vi "OptimizedFPGA_SPI_ReadAuto.vi"(8 "error in (no error)":errorcluster, 9 "Bytes per Sample":u32, 10 "Samples to Read":u32) -> (0 "error out":errorcluster, 2 "Data":u8[][](array[numeric]))   [LabVIEW 2017]
uses:
  <vilib>/Utility/error.llb/Error Cluster From Error Code.vi
  <vilib>/rvi/errors/niLvFpgaAdjustHostInterfaceError.vi
  <vilib>/rvi/interface/nirviMethod/nirviMethod.xnode
  <vilib>/Rock Robotics/SystemInterfaces/System/FPGA_SystemFRC FPGA Ref.ctl
  <vilib>/FPGAPlugInAG/Dynamic/niLvFpga_ReadFifo_Dynamic.vi
  <vilib>/rvi/errors/niLvFpgaMergeErrorWithErrorCode.vi
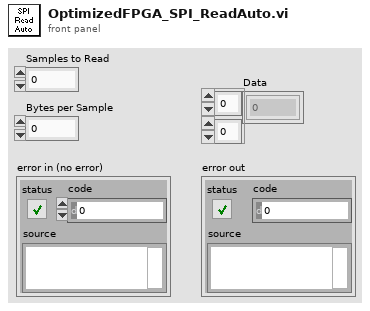
[diagram p1: front panel]
types:
  T1 = typedef "FPGA_SystemFRC FPGA Ref.ctl" = refnum<k20>
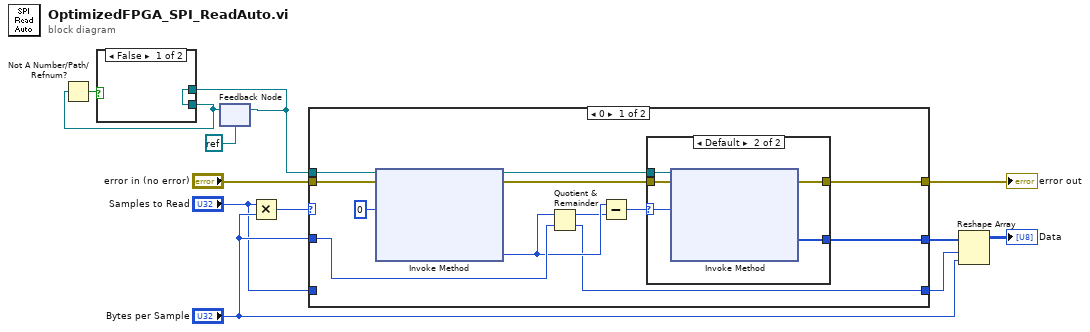
[diagram p0: block diagram]
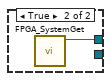
[diagram p2: hidden frame]
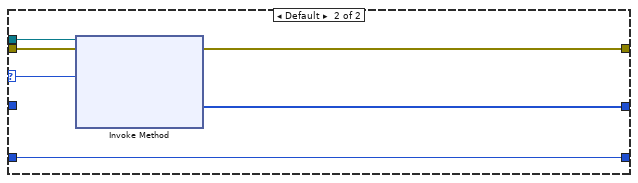
[diagram p4: hidden frame]
diagram:
  n1 = feedback #1(refnum<k0> refnum) -> (w2:T1)
  n2 = Not A Number/Path/Refnum?(number/path/refnum=w2) -> (NaN/Path/Refnum?=w3:bool)
  n3 = case shown="False" w3 {
    tunnel: [w13 w14] -> w4
    tunnel: w2 -> [w13 _]
    frame False {
    }
    frame True {
      n4 = call <vilib>:"FPGA_SystemGet.vi"() -> ("FRC FPGA Ref"=w14:T1)  [unwired: 11 in]
    }
  }
  n5 = feedback-in #1(w4) -> ()
  n6 = Multiply(x="Samples to Read", y="Bytes per Sample") -> (x*y=w9:u32)
  n7 = case shown="0" w9 {
    selector: w9 -> [_ w35]
    tunnel: [w21 w38] -> w12
    tunnel: "error in (no error)" -> [w26 w37]
    tunnel: w4 -> [w25 w36]
    tunnel: [w24 w34] -> w8
    tunnel: "Bytes per Sample" -> [w20 _]
    tunnel: [w15 w33] -> w5
    tunnel: "Samples to Read" -> [_ w33]
    frame 0 {
      n8 = xnode "Invoke Method"("FPGA VI Reference In"=w25, "error in"=w26, "Number of Elements"=u32 0) -> ("FPGA VI Reference Out"=w23:T1, "error out"=w22:errorcluster, "Elements Remaining"=w19:u32)  [unwired: 1 in, 1 out]
      n9 = Quotient & Remainder(x=w19, y=w20) -> (x-y*floor(x/y)=w18:u32, floor(x/y)=w15:u32)
      n10 = Subtract(x=w19, y=w18) -> (x-y=w17:u32)
      n11 = case shown="Default" w17 {
        selector: w17 -> [_ w29]
        tunnel: [_ w28] -> w24
        tunnel: w23 -> [_ w32]
        tunnel: w22 -> [w27 w31]
        tunnel: [w27 w30] -> w21
        frame 0 {
        }
        frame Default {
          n12 = xnode "Invoke Method"("FPGA VI Reference In"=w32, "error in"=w31, "Number of Elements"=w29) -> ("error out"=w30:errorcluster, "Data"=w28:u8[])  [unwired: 1 in, 2 out]
        }
      }
    }
    frame Default {
      n13 = xnode "Invoke Method"("FPGA VI Reference In"=w36, "error in"=w37, "Number of Elements"=w35) -> ("error out"=w38:errorcluster, "Data"=w34:u8[])  [unwired: 1 in, 2 out]
    }
  }
  "error out" <- w12
  n14 = Reshape Array(w8, w5, "Bytes per Sample") -> (→"Data":u8[][])
